vi "Close_Remote_Vi.vi"(4 "Also close host?":bool, 6 "Wait after host (ms)":u32, 8 "error in":errorcluster, 9 "Remote IP":string, 10 "Host Path":path, 11 "VI Path":path) -> (0 "error out":errorcluster)   [LabVIEW 2011]
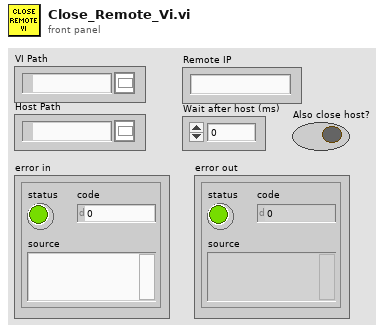
[diagram p1: front panel]
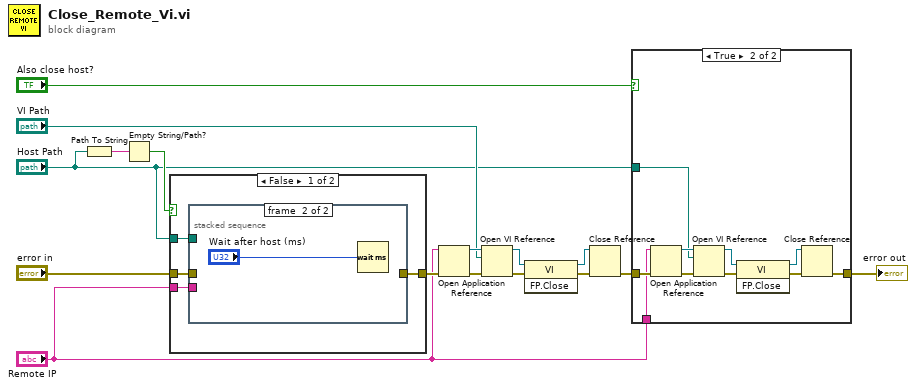
[diagram p0: block diagram]
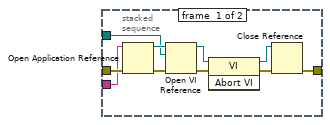
[diagram p3: hidden frame]
diagram:
  n1 = Path To String(path="Host Path") -> (string=w15:string)
  n2 = Empty String/Path?(string/path=w15) -> (empty?=w14:bool)
  n3 = case shown="False" w14 {
    tunnel: "error in" -> [w20 w32]
    tunnel: [w19 w32] -> w10
    tunnel: "Host Path" -> [w18 _]
    tunnel: "Remote IP" -> [w17 _]
    frame False {
      n4 = stacked-sequence {
        tunnel: w20 -> [w30 _]
        tunnel: [w23 _] -> w19
        tunnel: w18 -> [w22 _]
        tunnel: w17 -> [w21 _]
        frame #0 {
          n5 = Open Application Reference(8:w30, 11:w21) -> (0:w28:errorcluster, 3:w29:refnum<vi>)  [unwired: 2 in]
          n6 = Open VI Reference(application reference (local)=w29, vi path=w22, error in (no error)=w28) -> (vi reference=w26:refnum<vi>, error out=w27:errorcluster)  [unwired: 3 in]
          n7 = invoke class="VI" method="Abort VI"(reference=w26, error in=w27) -> (reference out=w24:refnum<vi>, error out=w25:errorcluster)  [unwired: 1 in, 1 out]
          n8 = Close Reference(reference=w24, error in (no error)=w25) -> (error out=w23:errorcluster)
        }
        frame #1 {
          n9 = Wait (ms)(milliseconds to wait="Wait after host (ms)") -> ()  [unwired: 1 out]
        }
      }
    }
    frame True {
    }
  }
  n10 = Open Application Reference(8:w10, 11:"Remote IP") -> (0:w13:errorcluster, 3:w12:refnum<vi>)  [unwired: 2 in]
  n11 = Open VI Reference(application reference (local)=w12, vi path="VI Path", error in (no error)=w13) -> (vi reference=w9:refnum<vi>, error out=w8:errorcluster)  [unwired: 3 in]
  n12 = invoke class="VI" method="FP.Close"(reference=w9, error in=w8) -> (reference out=w6:refnum<vi>, error out=w7:errorcluster)  [unwired: 1 in, 1 out]
  n13 = Close Reference(reference=w6, error in (no error)=w7) -> (error out=w4:errorcluster)
  n14 = case shown="True" "Also close host?" {
    tunnel: w4 -> [w33 w37]
    tunnel: [w33 w36] -> w3
    tunnel: "Host Path" -> [_ w35]
    tunnel: "Remote IP" -> [_ w34]
    frame False {
    }
    frame True {
      n15 = Open Application Reference(8:w37, 11:w34) -> (0:w38:errorcluster, 3:w39:refnum<vi>)  [unwired: 2 in]
      n16 = Open VI Reference(application reference (local)=w39, vi path=w35, error in (no error)=w38) -> (vi reference=w40:refnum<vi>, error out=w41:errorcluster)  [unwired: 3 in]
      n17 = invoke class="VI" method="FP.Close"(reference=w40, error in=w41) -> (reference out=w43:refnum<vi>, error out=w42:errorcluster)  [unwired: 1 in, 1 out]
      n18 = Close Reference(reference=w43, error in (no error)=w42) -> (error out=w36:errorcluster)
    }
  }
  "error out" <- w3
